vi "Receive Boolean Value Msg.vi"(8 "error in (no error)":errorcluster, 10 "BooleanValueMsg":refnum<class "BooleanValueMsg.lvclass">, 11 "AutoRegPanel In":refnum<class "AutoRegPanel.lvclass">) -> (0 "error out":errorcluster, 3 "AutoRegPanel Out":refnum<class "AutoRegPanel.lvclass">)   [LabVIEW 2015, in "TestActors.lvlib" / "AutoRegPanel.lvclass"]
uses:
  AutoRegPanel.lvclass
  AutoRegistration/ActorAutoRegistration Messages/BooleanValueMsg/BooleanValueMsg.lvclass
  IViewable/IViewable/IViewable.lvclass
  Dialog Box Implementations/OneButtonDialogBox/OneButtonDialogBox.lvclass
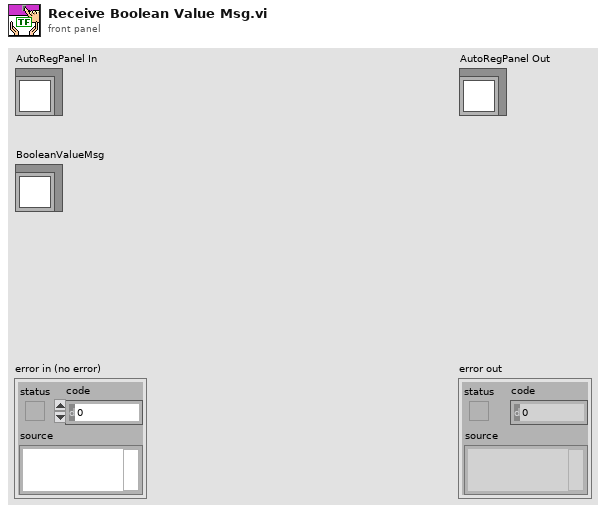
[diagram p1: front panel]
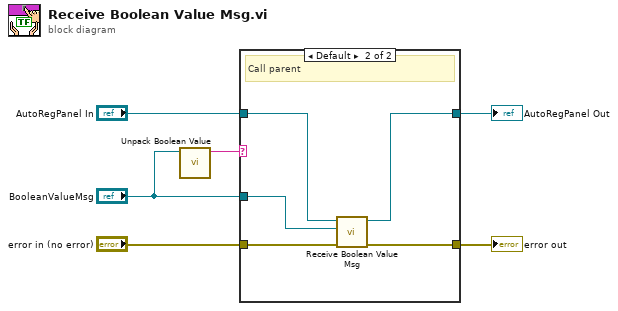
[diagram p0: block diagram]
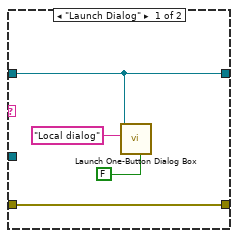
[diagram p2: hidden frame]
diagram:
  n1 = call-dynamic "Unpack Boolean Value.vi"("BooleanValueMsg in"="BooleanValueMsg") -> ("Name"=w1:string)  [unwired: 9 in, 1 out]
  n2 = case shown="Default" w1 {
    tunnel: [w10 w15] -> w6
    tunnel: [w9 w14] -> w5
    tunnel: "error in (no error)" -> [w10 w13]
    tunnel: "AutoRegPanel In" -> [w9 w12]
    tunnel: "BooleanValueMsg" -> [_ w11]
    frame "Launch Dialog" {
      n3 = call "Launch One-Button Dialog Box.vi"("Modal? (T)"=FALSE, "Message Text"="Local dialog", "Dialog Launcher"=w9) -> ()  [unwired: 8 in, 1 out]
    }
    frame Default {
      # "Call parent"
      n4 = call-parent "Receive Boolean Value Msg.vi"("error in (no error)"=w13, "BooleanValueMsg"=w11, "IViewable in"=w12) -> ("error out"=w15:errorcluster, "IViewable out"=w14:refnum<class "AutoRegPanel.lvclass">)  [unwired: 7 in]
    }
  }
  "error out" <- w6
  "AutoRegPanel Out" <- w5
